vi "osq_build.vi"(8 "error in":errorcluster, 11 "Sequencer Files":T1=[{"Sequence File"=path "Z:/Sequences/Energy Scan/Oct2014_200_5200.osq", "Repeats"=1, "Lines"=0}] caption="Sequencer Files (*.osq)" {"Repeats" min=1}) -> (0 "error out":errorcluster, 1 "Total Repeats":i32, 2 "SEQ":T2[](array[typedef]), 3 "Sequence Files":T1 {"Repeats" min=1}, 4 "Total Lines":i32, 7 "SEQ Files":path[](array[path]))   [LabVIEW 2015, in "oskar_tools.lvlib"]
uses:
  oskar_tools.lvlib
  seq_files.ctl
  seq_line.ctl
panel:
  in  "SEQ_Template":T2[](array[typedef])
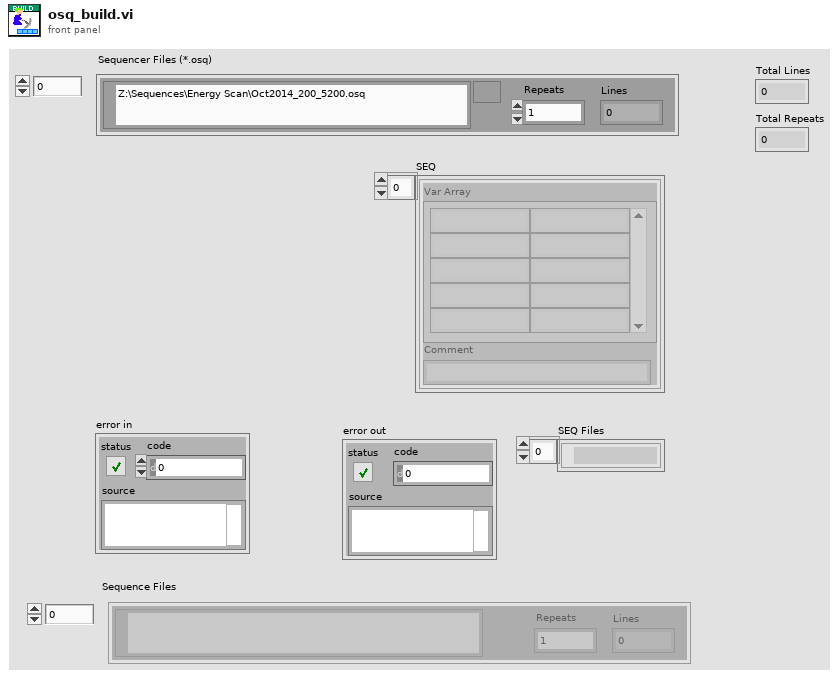
[diagram p1: front panel]
types:
  T1 = typedef "oskar_tools.lvlib/seq_files.ctl" = cluster{"Sequence File":path, "Repeats":i32, "Lines":i32}[]
  T2 = typedef "oskar_tools.lvlib/seq_line.ctl" = cluster{"Var Array":string[][], "Comment":string}
  T3 = cluster{"Sequence File":path, "Repeats":i32, "Lines":i32}
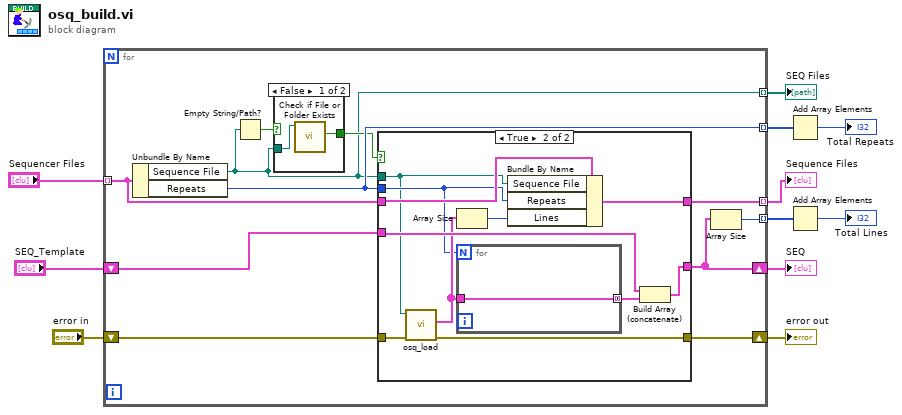
[diagram p0: block diagram]
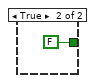
[diagram p2: hidden frame]
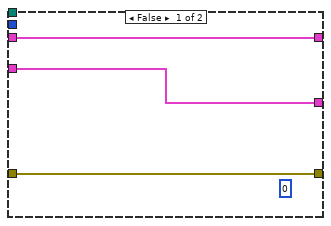
[diagram p3: hidden frame]
diagram:
  n1 = for {
    tunnel: "Sequencer Files" -> [w21] mode=indexing
    shift-right: [w13] -> w9
    shift-left: "SEQ_Template" -> [w22]
    tunnel: [w20] -> w8 mode=indexing
    tunnel: [w12] -> w7 mode=indexing
    tunnel: [w19] -> w5 mode=indexing
    shift-right: [w18] -> w2
    shift-left: "error in" -> [w17]
    tunnel: [w15] -> w1 mode=indexing
    n2 = Unbundle By Name(w21) -> ("Sequence File"=w15:path, "Repeats"=w19:i32)
    n3 = Empty String/Path?(string/path=w15) -> (empty?=w14:bool)
    n4 = case shown="False" w14 {
      tunnel: [w24 FALSE ("file or folder exists?")] -> w16
      tunnel: w15 -> [w23 _]
      frame False {
        n5 = call <vilib>:"Check if File or Folder Exists.vi"("path"=w23) -> ("file or folder exists?"=w24:bool)  [unwired: 8 in, 2 out]
      }
      frame True {
      }
    }
    n6 = case shown="True" w16 {
      tunnel: w22 -> [w27 w38]
      tunnel: [w27 w37] -> w13
      tunnel: w21 -> [w28 w35]
      tunnel: [w28 w34] -> w20
      tunnel: w19 -> [_ w32]
      tunnel: [w26 w31] -> w18
      tunnel: w17 -> [w26 w30]
      tunnel: w15 -> [_ w29]
      frame False {
        (unwired) 0
      }
      frame True {
        n7 = call "osq_load.vi"("error in (no error)"=w30, "Open"=w29) -> ("error out"=w31:errorcluster, "SEQs"=w36:T2[])  [unwired: 6 in, 2 out]
        n8 = Array Size(array=w36) -> (size(s)=w33:i32)
        n9 = for {
          N: w32 -> [_]
          tunnel: w36 -> [w40]
          tunnel: [w40] -> w39 mode=concatenating
        }
        n10 = Bundle By Name(cluster=w35, "Sequence File"=w29, "Repeats"=w32, "Lines"=w33) -> (w34:T3)
        n11 = Build Array (concatenate)(w38, w39) -> (w37:T2[])
      }
    }
    n12 = Array Size(array=w13) -> (size(s)=w12:i32)
  }
  "SEQ" <- w9
  "Sequence Files" <- w8
  "error out" <- w2
  "SEQ Files" <- w1
  n13 = Add Array Elements(numeric array=w5) -> (sum=→"Total Repeats":i32)
  n14 = Add Array Elements(numeric array=w7) -> (sum=→"Total Lines":i32)
